vi "analog latching relay.vi"(1 "RESET":bool, 2 "value":u32, 3 "READ":bool) -> (0 "out":u32)   [LabVIEW 2009]
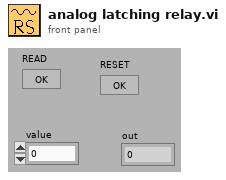
[diagram p1: front panel]
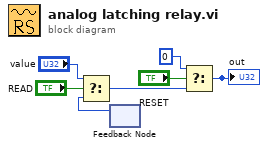
[diagram p0: block diagram]
diagram:
  n1 = feedback #1() -> (w1:u32)  [unwired: 1 in]
  n2 = Select(t="value", s="READ", f=w1) -> (s? t:f=w2:u32)
  n3 = Select(t=i16 0 ("in"), s="RESET", f=w2) -> (s? t:f=w7:u32)
  "out" <- w7
